vi "zadanie_2.vi"() -> ()   [LabVIEW 2020]
panel:
  out "Array 2":i32[][](array[numeric])
  out "Array":i32[][](array[numeric])
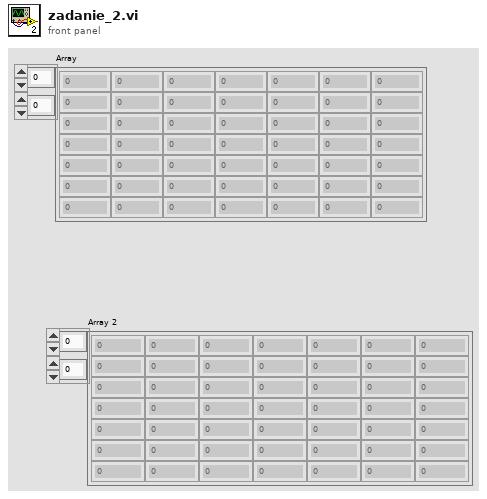
[diagram p1: front panel]
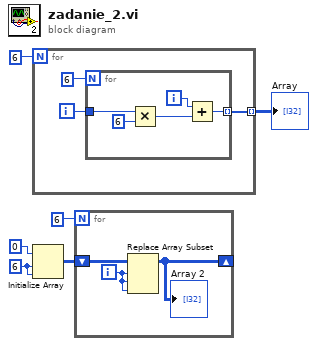
[diagram p0: block diagram]
diagram:
  w3 = 6 ("dimension size")
  n1 = for {
    N: 6 -> [_]
    tunnel: [w7] -> w5 mode=indexing
    i -> [w8]
    n2 = for {
      N: 6 -> [_]
      tunnel: w8 -> [w13]
      tunnel: [w10] -> w7 mode=indexing
      i -> [w11]
      n3 = Multiply(x=w13, y=6) -> (x*y=w12:i32)
      n4 = Add(x=w11, y=w12) -> (x+y=w10:i32)
    }
  }
  "Array" <- w5
  n5 = Initialize Array(0 ("element"), w3, w3) -> (w1:i32[][])
  n6 = for {
    N: 6 -> [_]
    shift-right: [w16] -> _
    shift-left: w1 -> [w17]
    i -> [w15]
    n7 = Replace Array Subset(array=w17, new element=w15, index (row)=w15, index (col)=w15) -> (w16:i32[][])
    "Array 2" <- w16
  }
